vi "host2.vi"() -> ()   [LabVIEW 2014]
uses:
  <vilib>/rvi/interface/nirviOpenFPGA/nirviOpenFPGA.xnode
  <vilib>/rvi/interface/nirviCloseFPGA/nirviCloseFPGA.xnode
  <vilib>/rvi/interface/nirviMethod/nirviMethod.xnode
  <vilib>/FPGAPlugInAG/Dynamic/niLvFpga_ReadFifo_Dynamic.vi
  <vilib>/rvi/errors/niLvFpgaMergeErrorWithErrorCode.vi
  <vilib>/FPGAPlugInAG/Dynamic/niLvFpga_StopFifo_Dynamic.vi
  <vilib>/FPGAPlugInAG/Dynamic/niLvFpga_WriteFifo_Dynamic.vi
  <vilib>/FPGAPlugInAG/Dynamic/niLvFpga_ConfigureFifo_Dynamic.vi
  <vilib>/FPGAPlugInAG/Dynamic/niLvFpga_StartFifo_Dynamic.vi
  <vilib>/rvi/interface/nirviReadWriteControl/nirviReadWriteControl.xnode
  <vilib>/ptbypt/NI_PtbyPt.lvlib
  <vilib>/FPGAPlugInAG/Dynamic/niLvFpga_Reset_Dynamic.vi
  <vilib>/FPGAPlugInAG/Dynamic/niLvFpga_Run_Dynamic.vi
  NiFpgaLv.dll
  <vilib>/Utility/error.llb/Error Cluster From Error Code.vi
  <vilib>/rvi/interface/Simulation/niFpgaSimulationCallBeginRW.vi
  <vilib>/rvi/errors/niLvFpgaAdjustHostInterfaceError.vi
  <vilib>/FPGAPlugInAG/Dynamic/niLvFpga_Close_Dynamic.vi
  target.vi
panel:
  in  "gain":i16
  out "fft rx":dbl[](graph)
  out "fft tx":dbl[](graph)
  out "wf tx":dbl[][](graph)
  out "wf rx":dbl[][](graph)
  out "EVM (%)":dbl format="%#_6f"
  out "MER (dB)":dbl
  in  "noise":bool
  in  "standard deviation":dbl(slide)=1.0 min=0.0 max=500.0 step=5.0 scale=0.5..500.0
  out "rx":cluster{dbl[], dbl[]}[](graph)
  out "tx":cluster{dbl[], dbl[]}[](graph)
  in  "stop":bool
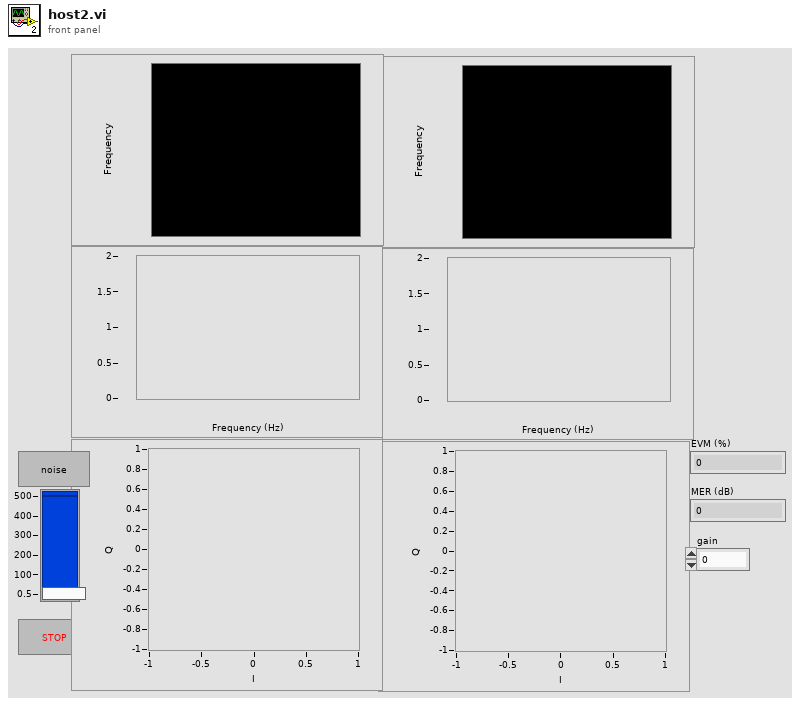
[diagram p1: front panel]
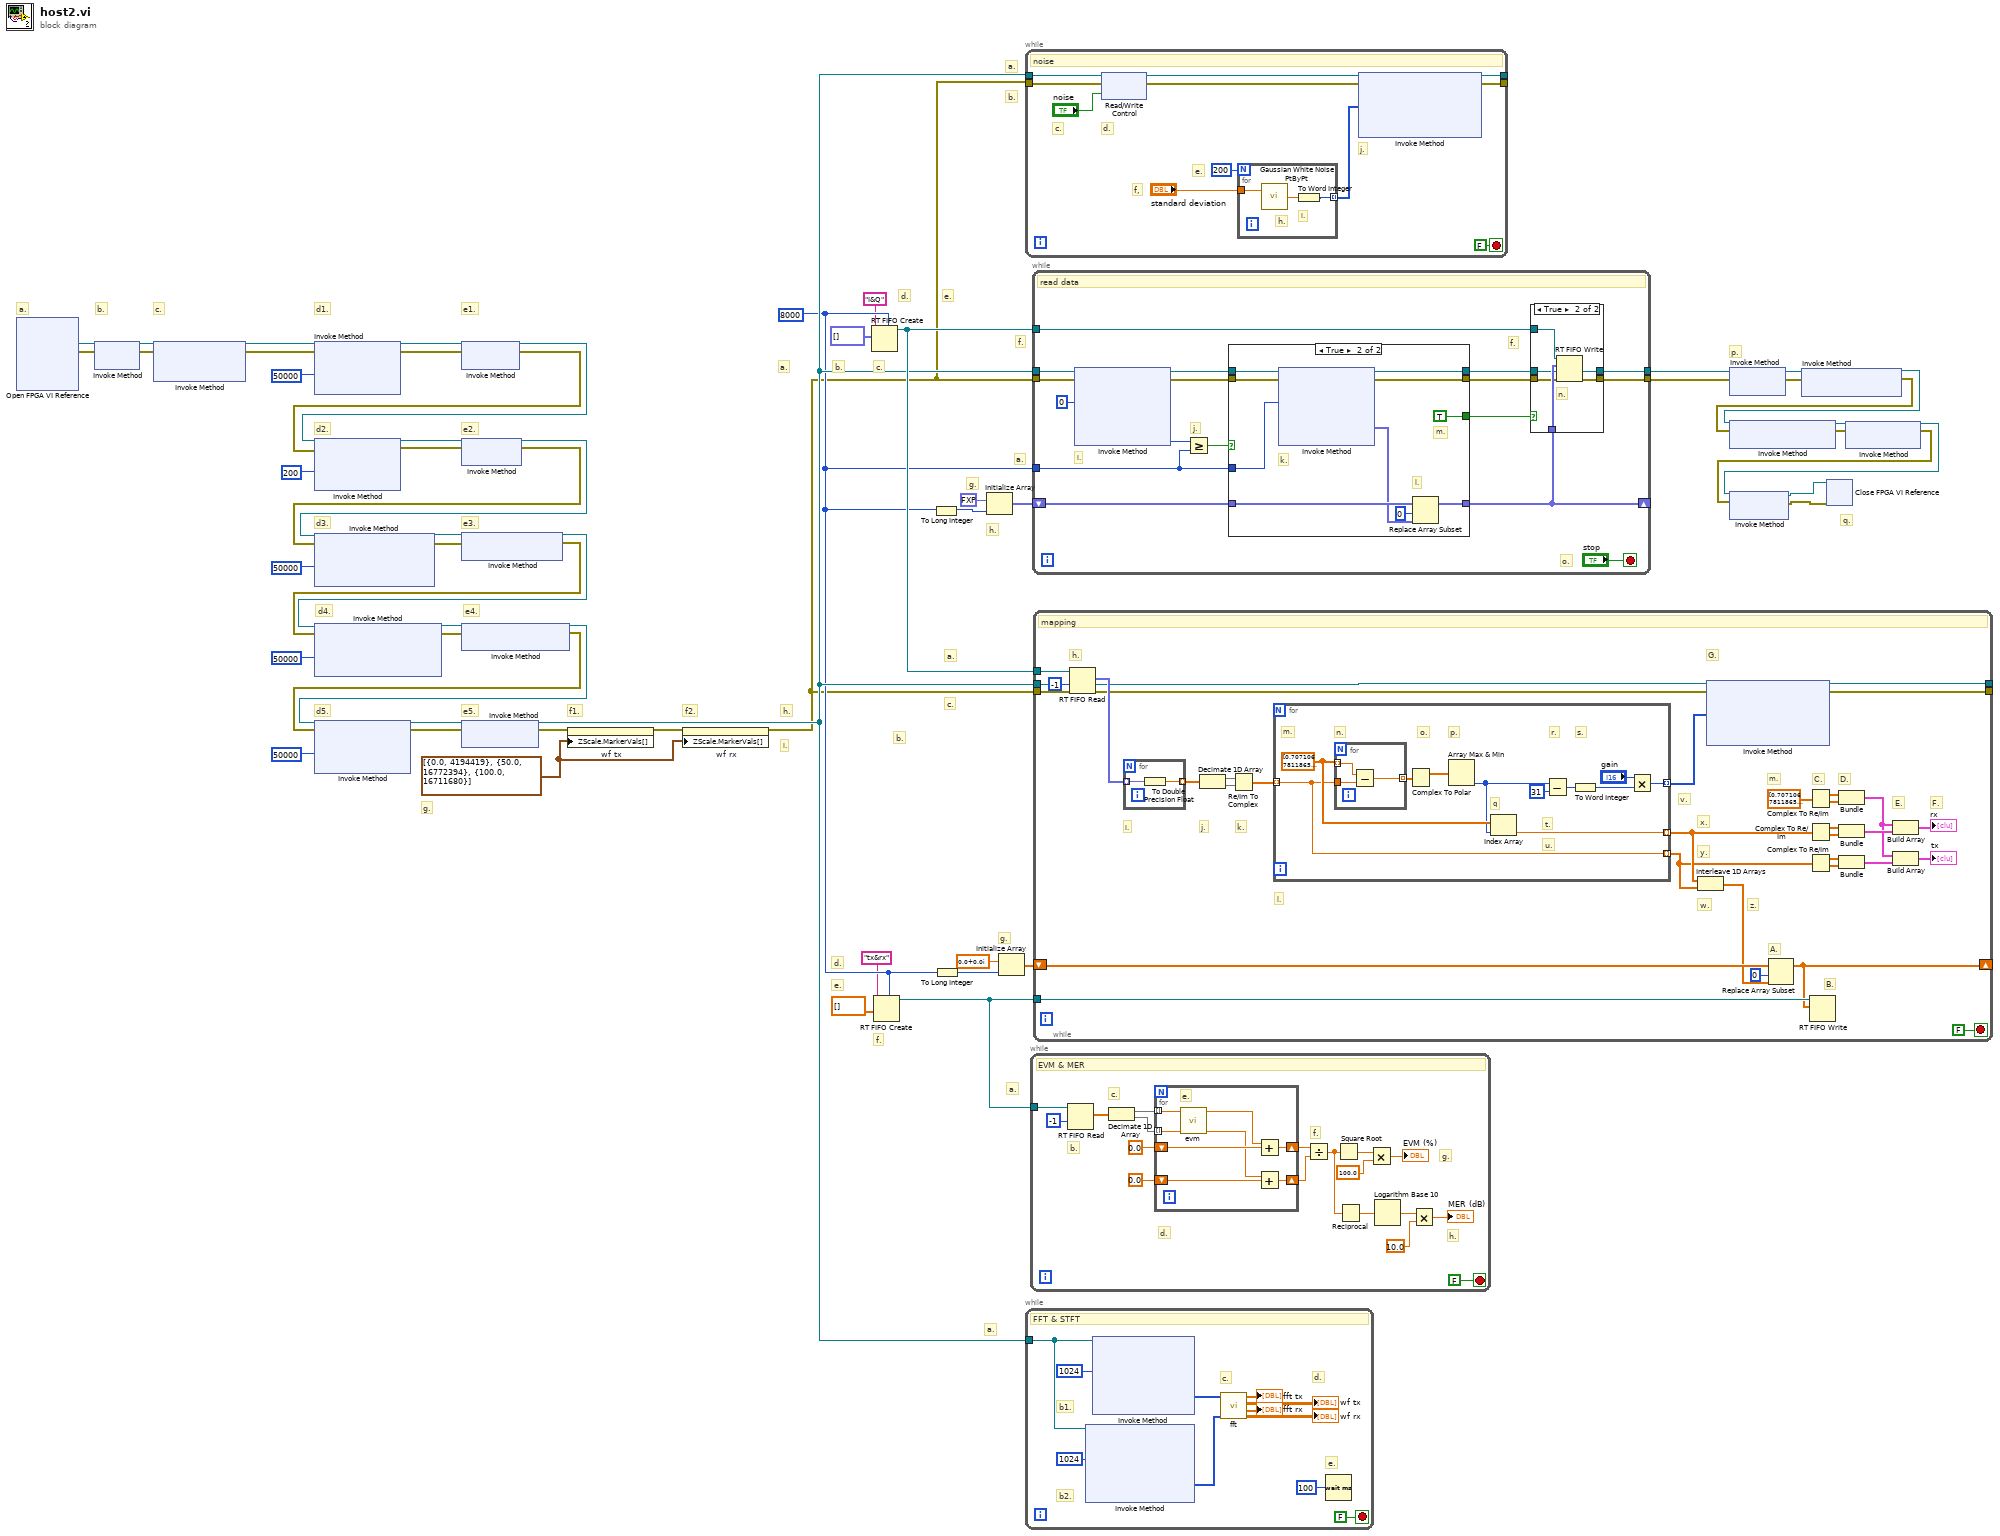
[diagram p0: block diagram]
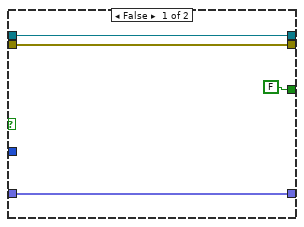
[diagram p3: hidden frame]
diagram:
  w15 = u32 8000 ("elements to read FIFO")
  w14 = cluster{dbl, u32}[] [{0.0, 4194419}, {50.0, 16772394}, {100.0, 16711680}] ("Z Scale.Marker Values[]")
  # "a."
  # "a."
  # "g."
  # "f."
  # "e."
  # "d."
  # "c."
  # "b."
  # "a."
  # "i."
  # "h."
  # "g."
  # "f2."
  # "f1."
  # "e5."
  # "d5."
  # "e4."
  # "d4."
  # "e3."
  # "d3."
  # "e2."
  # "d2."
  # "e1."
  # "d1."
  # "c."
  # "b."
  # "a."
  # "q."
  # "p."
  # "h."
  # "g."
  # "a."
  # "f."
  # "e."
  # "d."
  # "c."
  # "b."
  # "a."
  # "b."
  # "a."
  n1 = xnode "Open FPGA VI Reference"() -> ("FPGA VI Reference Out"=w25:refnum<k20>, "error out"=w24:errorcluster)  [unwired: 2 in]
  n2 = xnode "Invoke Method"("FPGA VI Reference In"=w25, "error in"=w24) -> ("FPGA VI Reference Out"=w23:refnum<k20>, "error out"=w22:errorcluster)
  n3 = xnode "Invoke Method"("FPGA VI Reference In"=w23, "error in"=w22) -> ("FPGA VI Reference Out"=w21:refnum<k20>, "error out"=w20:errorcluster)  [unwired: 1 in]
  n4 = xnode "Invoke Method"("FPGA VI Reference In"=w21, "error in"=w20, "Requested Depth"=u32 50000) -> ("FPGA VI Reference Out"=w53:refnum<k20>, "error out"=w54:errorcluster)  [unwired: 1 out]
  n5 = xnode "Invoke Method"("FPGA VI Reference In"=w53, "error in"=w54) -> ("FPGA VI Reference Out"=w35:refnum<k20>, "error out"=w36:errorcluster)
  n6 = xnode "Invoke Method"("FPGA VI Reference In"=w35, "error in"=w36, "Requested Depth"=u32 200) -> ("FPGA VI Reference Out"=w33:refnum<k20>, "error out"=w34:errorcluster)  [unwired: 1 out]
  n7 = xnode "Invoke Method"("FPGA VI Reference In"=w33, "error in"=w34) -> ("FPGA VI Reference Out"=w31:refnum<k20>, "error out"=w32:errorcluster)
  n8 = xnode "Invoke Method"("FPGA VI Reference In"=w31, "error in"=w32, "Requested Depth"=u32 50000) -> ("FPGA VI Reference Out"=w52:refnum<k20>, "error out"=w51:errorcluster)  [unwired: 1 out]
  n9 = xnode "Invoke Method"("FPGA VI Reference In"=w52, "error in"=w51) -> ("FPGA VI Reference Out"=w41:refnum<k20>, "error out"=w42:errorcluster)
  n10 = xnode "Invoke Method"("FPGA VI Reference In"=w41, "error in"=w42, "Requested Depth"=u32 50000) -> ("FPGA VI Reference Out"=w43:refnum<k20>, "error out"=w44:errorcluster)  [unwired: 1 out]
  n11 = xnode "Invoke Method"("FPGA VI Reference In"=w43, "error in"=w44) -> ("FPGA VI Reference Out"=w39:refnum<k20>, "error out"=w40:errorcluster)
  n12 = xnode "Invoke Method"("FPGA VI Reference In"=w39, "error in"=w40, "Requested Depth"=u32 50000) -> ("FPGA VI Reference Out"=w50:refnum<k20>, "error out"=w49:errorcluster)  [unwired: 1 out]
  n13 = xnode "Invoke Method"("FPGA VI Reference In"=w50, "error in"=w49) -> ("FPGA VI Reference Out"=w30:refnum<k20>, "error out"=w4:errorcluster)
  n14 = property on="wf tx" class="IntChart (strict)"(error in=w4, "ZScale.MarkerVals[]"=w14) -> (error out=w5:errorcluster)  [unwired: 1 in, 1 out]
  n15 = property on="wf rx" class="IntChart (strict)"(error in=w5, "ZScale.MarkerVals[]"=w14) -> (error out=w3:errorcluster)  [unwired: 1 in, 1 out]
  n16 = RT FIFO Create(0:"I&Q" ("name (unnamed)"), 1:fxp<+/-,20,4>[] [], 6:w15) -> (8:w55:refnum<k33>)  [unwired: 5 in, 2 out]
  n17 = RT FIFO Create(0:"tx&rx" ("name (unnamed)"), 1:cdb[] [], 6:w15) -> (8:w16:refnum<k33>)  [unwired: 5 in, 2 out]
  n18 = To Long Integer(number=w15) -> (32bit integer=w7:i32)
  n19 = To Long Integer(number=w15) -> (32bit integer=w6:i32)
  n20 = Initialize Array(fxp<+/-,20,4> 0.0, w7) -> (w59:fxp<+/-,20,4>[])
  n21 = Initialize Array(cdb 0.0+0.0i, w6) -> (w17:cdb[])
  n22 = while {
    tunnel: w30 -> [w69]
    tunnel: w3 -> [w63]
    tunnel: [w67] -> _
    tunnel: [w66] -> _
    stop <- FALSE stop-if-true
    # "j."
    # "f,"
    # "e."
    # "d."
    # "c."
    # "noise"
    n23 = xnode "Read/Write Control"("FPGA VI Reference In"=w69, "error in"=w63, "noise"="noise") -> ("error out"=w68:errorcluster)  [unwired: 1 out]
    n24 = for {
      N: 200 ("samples") -> [_]
      tunnel: "standard deviation" -> [w72]
      tunnel: [w70] -> w60 mode=indexing
      # "i."
      # "h."
      n25 = call <vilib>:"Gaussian White Noise PtByPt.vi"("standard deviation"=w72) -> ("Gaussian white noise"=w71:dbl)  [unwired: 2 in]
      n26 = To Word Integer(number=w71) -> (16bit integer=w70:i16)
    }
    n27 = xnode "Invoke Method"("FPGA VI Reference In"=w69, "error in"=w68, "Data"=w60) -> ("FPGA VI Reference Out"=w66:refnum<k20>, "error out"=w67:errorcluster)  [unwired: 1 in, 1 out]
  }
  n28 = while {
    tunnel: w30 -> [w83]
    stop <- FALSE stop-if-true
    # "e."
    # "d."
    # "c."
    # "b2."
    # "b1."
    # "FFT & STFT"
    n29 = xnode "Invoke Method"("FPGA VI Reference In"=w83, "Number of Elements"=u32 1024) -> ("Data"=w80:i8[])  [unwired: 2 in, 3 out]
    n30 = xnode "Invoke Method"("FPGA VI Reference In"=w83, "Number of Elements"=u32 1024) -> ("Data"=w81:i8[])  [unwired: 2 in, 3 out]
    n31 = call "fft.vi"("rx"=w80, "tx"=w81) -> ("wf rx"=→"wf rx":dbl[][], "fft rx"=→"fft rx":dbl[], "wf tx"=→"wf tx":dbl[][], "fft tx"=→"fft tx":dbl[])  [unwired: 6 in]
    n32 = Wait (ms)(milliseconds to wait=u32 100) -> ()  [unwired: 1 out]
  }
  n33 = while {
    tunnel: w16 -> [w101]
    stop <- FALSE stop-if-true
    # "h."
    # "g."
    # "f."
    # "d."
    # "c."
    # "b."
    # "EVM & MER"
    n34 = RT FIFO Read(0:w101, 2:-1 ("timeout in ms (0)")) -> (9:w99:cdb[])  [unwired: 2 in, 4 out]
    n35 = Decimate 1D Array(w99) -> (w98:cdb[], w97:cdb[])
    n36 = for {
      tunnel: w98 -> [w109] mode=indexing
      tunnel: w97 -> [w108] mode=indexing
      shift-right: [w105] -> w91
      shift-left: 0.0 -> [w106]
      shift-right: [w102] -> w90
      shift-left: 0.0 -> [w103]
      # "e."
      n37 = call "evm.vi"("rx"=w108, "tx"=w109) -> ("den"=w104:dbl, "num"=w107:dbl)  [unwired: 8 in]
      n38 = Add(x=w107, y=w106) -> (x+y=w105:dbl)
      n39 = Add(x=w104, y=w103) -> (x+y=w102:dbl)
    }
    n40 = Divide(x=w91, y=w90) -> (x/y=w88:dbl)
    n41 = Square Root(x=w88) -> (sqrt(x)=w94:dbl)
    n42 = Reciprocal(x=w88) -> (1/x=w87:dbl)
    n43 = Multiply(x=w94, y=100.0) -> (x*y=→"EVM (%)":dbl)
    n44 = Logarithm Base 10(1:w87) -> (0:w86:dbl)
    n45 = Multiply(x=w86, y=10.0) -> (x*y=→"MER (dB)":dbl)
  }
  n46 = while {
    shift-right: [w124] -> _
    shift-left: w59 -> [w125]
    tunnel: w55 -> [w123]
    tunnel: [w115] -> w8
    tunnel: w30 -> [w119]
    tunnel: w3 -> [w118]
    tunnel: [w113] -> w56
    tunnel: w15 -> [w122]
    stop <- "stop" stop-if-true
    # "o."
    # "f."
    # "j."
    # "i."
    # "read data"
    n47 = xnode "Invoke Method"("FPGA VI Reference In"=w119, "error in"=w118, "Number of Elements"=u32 0) -> ("FPGA VI Reference Out"=w121:refnum<k20>, "error out"=w120:errorcluster, "Elements Remaining"=w116:u32)  [unwired: 1 in, 1 out]
    n48 = Greater Or Equal?(x=w116, y=w122) -> (x >= y?=w126:bool)
    n49 = case shown="True" w126 {
      tunnel: w121 -> [w136 w142]
      tunnel: w120 -> [w135 w147]
      tunnel: w122 -> [_ w140]
      tunnel: w125 -> [w137 w146]
      tunnel: [w137 w145] -> w124
      tunnel: [w136 w144] -> w112
      tunnel: [w135 w143] -> w110
      tunnel: [FALSE TRUE] -> w111
      frame False {
      }
      frame True {
        # "m."
        # "l."
        # "k."
        n50 = xnode "Invoke Method"("FPGA VI Reference In"=w142, "error in"=w147, "Number of Elements"=w140) -> ("FPGA VI Reference Out"=w144:refnum<k20>, "error out"=w143:errorcluster, "Data"=w141:fxp<+/-,20,4>[])  [unwired: 1 in, 1 out]
        n51 = Replace Array Subset(array=w146, new element=w141, index=0) -> (w145:fxp<+/-,20,4>[])
      }
    }
    n52 = case shown="True" w111 {
      tunnel: w124 -> [_ w133]
      tunnel: w123 -> [_ w132]
      tunnel: w110 -> [w128 w131]
      tunnel: [w128 w130] -> w115
      tunnel: [w127 w129] -> w113
      tunnel: w112 -> [w127 w129]
      frame False {
      }
      frame True {
        # "n."
        n53 = RT FIFO Write(0:w132, 1:w133, 3:w131) -> (11:w130:errorcluster)  [unwired: 2 in, 3 out]
      }
    }
  }
  n54 = while {
    tunnel: w55 -> [w180]
    tunnel: w3 -> [w172]
    tunnel: w30 -> [w176]
    tunnel: w16 -> [w167]
    shift-right: [w166] -> _
    shift-left: w17 -> [w169]
    tunnel: [w161] -> _
    tunnel: [w160] -> _
    stop <- FALSE stop-if-true
    # "G."
    # "F."
    # "E."
    # "D."
    # "C."
    # "m."
    # "B."
    # "A."
    # "z."
    # "w."
    # "y."
    # "x."
    # "v."
    # "l."
    # "k."
    # "j."
    # "i."
    # "h."
    # "mapping"
    n55 = RT FIFO Read(0:w180, 2:-1 ("timeout in ms (0)"), 3:w172) -> (9:w177:fxp<+/-,20,4>[], 11:w171:errorcluster)  [unwired: 1 in, 3 out]
    n56 = for {
      tunnel: w177 -> [w182] mode=indexing
      tunnel: [w181] -> w178 mode=indexing
      n57 = To Double Precision Float(number=w182) -> (double precision float=w181:dbl)
    }
    n58 = Decimate 1D Array(w178) -> (w175:dbl[], w174:dbl[])
    n59 = Re/Im To Complex(1:w174, 2:w175) -> (0:w173:cdb[])
    n60 = for {
      tunnel: [w184] -> w165 mode=indexing
      tunnel: w173 -> [w186] mode=indexing
      tunnel: [w186] -> w163 mode=indexing
      tunnel: [w187] -> w164 mode=indexing
      w189 = cdb[] [0.7071067811865476+0.7071067811865476i, 0.5050762722761054+0.7071067811865476i, 0.10101525445522107+0.7071067811865476i, 0.30304576336566325+0.7071067811865476i, -0.7071067811865476+0.7071067811865476i, -0.5050762722761054+0.7071067811865476i, -0.10101525445522107+0.7071067811865476i, -0.30304576336566325+0.7071067811865476i, 0.7071067811865476+0.5050762722761054i, 0.5050762722761054+0.5050762722761054i, 0.10101525445522107+0.5050762722761054i, 0.30304576336566325+0.5050762722761054i, -0.7071067811865476+0.5050762722761054i, -0.5050762722761054+0.5050762722761054i, -0.10101525445522107+0.5050762722761054i, -0.30304576336566325+0.5050762722761054i, 0.7071067811865476+0.10101525445522107i, 0.5050762722761054+0.10101525445522107i, 0.10101525445522107+0.10101525445522107i, 0.30304576336566325+0.10101525445522107i, -0.7071067811865476+0.10101525445522107i, -0.5050762722761054+0.10101525445522107i, -0.10101525445522107+0.10101525445522107i, -0.30304576336566325+0.10101525445522107i, 0.7071067811865476+0.30304576336566325i, 0.5050762722761054+0.30304576336566325i, 0.10101525445522107+0.30304576336566325i, 0.30304576336566325+0.30304576336566325i, -0.7071067811865476+0.30304576336566325i, -0.5050762722761054+0.30304576336566325i, -0.10101525445522107+0.30304576336566325i, -0.30304576336566325+0.30304576336566325i, 0.7071067811865476-0.7071067811865476i, 0.5050762722761054-0.7071067811865476i, 0.10101525445522107-0.7071067811865476i, 0.30304576336566325-0.7071067811865476i, -0.7071067811865476-0.7071067811865476i, -0.5050762722761054-0.7071067811865476i, -0.10101525445522107-0.7071067811865476i, -0.30304576336566325-0.7071067811865476i, 0.7071067811865476-0.5050762722761054i, 0.5050762722761054-0.5050762722761054i, 0.10101525445522107-0.5050762722761054i, 0.30304576336566325-0.5050762722761054i, -0.7071067811865476-0.5050762722761054i, -0.5050762722761054-0.5050762722761054i, -0.10101525445522107-0.5050762722761054i, -0.30304576336566325-0.5050762722761054i, 0.7071067811865476-0.10101525445522107i, 0.5050762722761054-0.10101525445522107i, 0.10101525445522107-0.10101525445522107i, 0.30304576336566325-0.10101525445522107i, -0.7071067811865476-0.10101525445522107i, -0.5050762722761054-0.10101525445522107i, -0.10101525445522107-0.10101525445522107i, -0.30304576336566325-0.10101525445522107i, 0.7071067811865476-0.30304576336566325i, 0.5050762722761054-0.30304576336566325i, 0.10101525445522107-0.30304576336566325i, 0.30304576336566325-0.30304576336566325i, -0.7071067811865476-0.30304576336566325i, -0.5050762722761054-0.30304576336566325i, -0.10101525445522107-0.30304576336566325i, -0.30304576336566325-0.30304576336566325i] ("symbol map")
      # "u."
      # "t."
      # "s."
      # "r."
      # "q"
      # "p."
      # "o."
      # "n."
      # "m."
      n61 = for {
        tunnel: w189 -> [w196] mode=indexing
        tunnel: [w195] -> w190 mode=indexing
        tunnel: w186 -> [w194]
        n62 = Subtract(x=w196, y=w194) -> (x-y=w195:cdb)
      }
      n63 = Complex To Polar(r * e^(i*theta)=w190) -> (r=w193:dbl[])  [unwired: 1 out]
      n64 = Array Max & Min(array=w193) -> (min index (indices)=w188:i32)  [unwired: 3 out]
      n65 = Index Array(array=w189, index=w188) -> (element=w187:cdb)
      n66 = Subtract(x=w188, y=31) -> (x-y=w191:i32)
      n67 = To Word Integer(number=w191) -> (16bit integer=w185:i16)
      n68 = Multiply(x="gain", y=w185) -> (x*y=w184:i16)
    }
    n69 = Interleave 1D Arrays(w164, w163) -> (w162:cdb[])
    n70 = xnode "Invoke Method"("FPGA VI Reference In"=w176, "error in"=w171, "Data"=w165) -> ("FPGA VI Reference Out"=w160:refnum<k20>, "error out"=w161:errorcluster)  [unwired: 1 in, 1 out]
    n71 = Replace Array Subset(array=w169, new element=w162, index=0) -> (w166:cdb[])
    n72 = Complex To Re/Im(x + iy=cdb[] [0.7071067811865476+0.7071067811865476i, 0.5050762722761054+0.7071067811865476i, 0.10101525445522107+0.7071067811865476i, 0.30304576336566325+0.7071067811865476i, -0.7071067811865476+0.7071067811865476i, -0.5050762722761054+0.7071067811865476i, -0.10101525445522107+0.7071067811865476i, -0.30304576336566325+0.7071067811865476i, 0.7071067811865476+0.5050762722761054i, 0.5050762722761054+0.5050762722761054i, 0.10101525445522107+0.5050762722761054i, 0.30304576336566325+0.5050762722761054i, -0.7071067811865476+0.5050762722761054i, -0.5050762722761054+0.5050762722761054i, -0.10101525445522107+0.5050762722761054i, -0.30304576336566325+0.5050762722761054i, 0.7071067811865476+0.10101525445522107i, 0.5050762722761054+0.10101525445522107i, 0.10101525445522107+0.10101525445522107i, 0.30304576336566325+0.10101525445522107i, -0.7071067811865476+0.10101525445522107i, -0.5050762722761054+0.10101525445522107i, -0.10101525445522107+0.10101525445522107i, -0.30304576336566325+0.10101525445522107i, 0.7071067811865476+0.30304576336566325i, 0.5050762722761054+0.30304576336566325i, 0.10101525445522107+0.30304576336566325i, 0.30304576336566325+0.30304576336566325i, -0.7071067811865476+0.30304576336566325i, -0.5050762722761054+0.30304576336566325i, -0.10101525445522107+0.30304576336566325i, -0.30304576336566325+0.30304576336566325i, 0.7071067811865476-0.7071067811865476i, 0.5050762722761054-0.7071067811865476i, 0.10101525445522107-0.7071067811865476i, 0.30304576336566325-0.7071067811865476i, -0.7071067811865476-0.7071067811865476i, -0.5050762722761054-0.7071067811865476i, -0.10101525445522107-0.7071067811865476i, -0.30304576336566325-0.7071067811865476i, 0.7071067811865476-0.5050762722761054i, 0.5050762722761054-0.5050762722761054i, 0.10101525445522107-0.5050762722761054i, 0.30304576336566325-0.5050762722761054i, -0.7071067811865476-0.5050762722761054i, -0.5050762722761054-0.5050762722761054i, -0.10101525445522107-0.5050762722761054i, -0.30304576336566325-0.5050762722761054i, 0.7071067811865476-0.10101525445522107i, 0.5050762722761054-0.10101525445522107i, 0.10101525445522107-0.10101525445522107i, 0.30304576336566325-0.10101525445522107i, -0.7071067811865476-0.10101525445522107i, -0.5050762722761054-0.10101525445522107i, -0.10101525445522107-0.10101525445522107i, -0.30304576336566325-0.10101525445522107i, 0.7071067811865476-0.30304576336566325i, 0.5050762722761054-0.30304576336566325i, 0.10101525445522107-0.30304576336566325i, 0.30304576336566325-0.30304576336566325i, -0.7071067811865476-0.30304576336566325i, -0.5050762722761054-0.30304576336566325i, -0.10101525445522107-0.30304576336566325i, -0.30304576336566325-0.30304576336566325i] ("symbol map")) -> (x=w154:dbl[], y=w153:dbl[])
    n73 = Complex To Re/Im(x + iy=w164) -> (x=w159:dbl[], y=w158:dbl[])
    n74 = Complex To Re/Im(x + iy=w163) -> (x=w157:dbl[], y=w156:dbl[])
    n75 = RT FIFO Write(0:w167, 1:w166) -> ()  [unwired: 3 in, 4 out]
    n76 = Bundle(w154, w153) -> (w151:cluster{dbl[], dbl[]})  [unwired: 1 in]
    n77 = Bundle(w159, w158) -> (w152:cluster{dbl[], dbl[]})  [unwired: 1 in]
    n78 = Bundle(w157, w156) -> (w150:cluster{dbl[], dbl[]})  [unwired: 1 in]
    n79 = Build Array(w151, w152) -> (→"rx":cluster{dbl[], dbl[]}[])
    n80 = Build Array(w151, w150) -> (→"tx":cluster{dbl[], dbl[]}[])
  }
  n81 = xnode "Invoke Method"("FPGA VI Reference In"=w56, "error in"=w8) -> ("FPGA VI Reference Out"=w48:refnum<k20>, "error out"=w46:errorcluster)
  n82 = xnode "Invoke Method"("FPGA VI Reference In"=w48, "error in"=w46) -> ("FPGA VI Reference Out"=w47:refnum<k20>, "error out"=w45:errorcluster)
  n83 = xnode "Invoke Method"("FPGA VI Reference In"=w47, "error in"=w45) -> ("FPGA VI Reference Out"=w38:refnum<k20>, "error out"=w37:errorcluster)
  n84 = xnode "Invoke Method"("FPGA VI Reference In"=w38, "error in"=w37) -> ("FPGA VI Reference Out"=w28:refnum<k20>, "error out"=w29:errorcluster)
  n85 = xnode "Invoke Method"("FPGA VI Reference In"=w28, "error in"=w29) -> ("FPGA VI Reference Out"=w27:refnum<k20>, "error out"=w26:errorcluster)
  n86 = xnode "Close FPGA VI Reference"("FPGA VI Reference In"=w27, "error in"=w26) -> ()  [unwired: 1 out]
